vi "Do.vi"(8 "error in (no error)":errorcluster, 10 "Actor in":refnum<class "Actor.lvclass">, 11 "Update Energy Storage Parameter Msg":refnum<class "Update Energy Storage Parameter Msg.lvclass">) -> (0 "error out":errorcluster, 2 "Actor out":refnum<class "Actor.lvclass">)   [LabVIEW 2016, in "Optimization Framework.lvlib" / "Update Energy Storage Parameter Msg.lvclass"]
doc: "This VI delivers the message to the actor by calling the appropriate method(s) on the actor."
uses:
  Update Energy Storage Parameter Msg.lvclass
  <vilib>/ActorFramework/Actor/Actor.lvclass
  Optimization/Optimization.lvclass
  C:/Program Files (x86)/National Instruments/LabVIEW 2016/vi.lib/ActorFramework/Actor/Actor.lvclass
  Update Energy Storage Parameter Msg.lvclass/Update Energy Storage Parameter Msg.ctl
  Optimization/Optimization.lvclass/Optimization.ctl
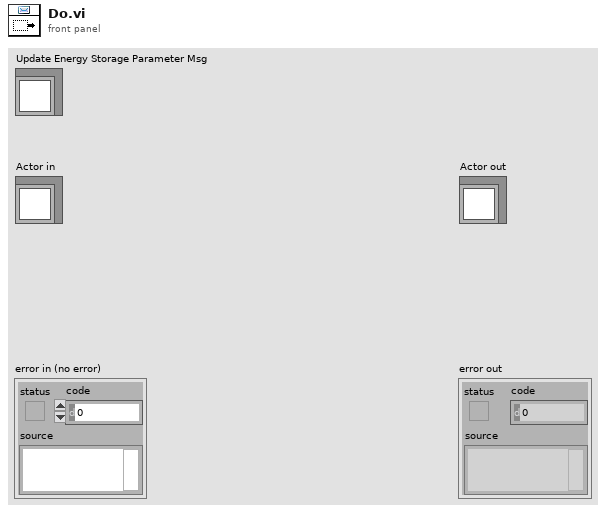
[diagram p1: front panel]
types:
  T1 = typedef "Optimization Framework.lvlib/Optimization.lvclass/Optimization Parameters Energy Storage.ctl" = cluster{"Device ID":u64, "Bus ID":u16, "Voltage (V)":dbl, "Power Rating (kVA)":dbl, "Energy Rating (kWh)":dbl, "Ramp Rate (kW/s)":dbl, "Max Power Factor (leading)":dbl, "Max Power Factor (lagging)":dbl, "Charging Efficiency Curve Power":dbl[], "Charging Efficiency Curve Efficiency":dbl[], "Discharging Efficiency Curve Power":dbl[], "Discharging Efficiency Curve Efficiency":dbl[], "Min SOC(%)":dbl, "Max SOC(%)":dbl, "Start SOC(%)":dbl, "End SOC(%)":dbl, "Control Capabilities":T2}
  T2 = typedef "Optimization Framework.lvlib/Optimization.lvclass/Device Control Capabilities.ctl" = cluster{"VF":bool, "P":bool, "Q":bool, "PF":bool, "PV":bool}
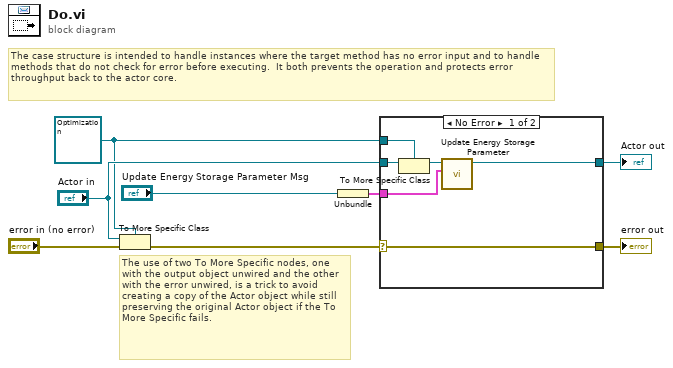
[diagram p0: block diagram]
diagram:
  w2 = refnum<class "Optimization.lvclass"> refnum ("Actor in")
  # "The use of two To More Specific nodes, one with the output object unwired and the other with the error unwired, is a trick to avoid creating a copy of the Actor object while still preserving the original Actor object if the To More Specific fails."
  # "The case structure is intended to handle instances where the target method has no error input and to handle methods that do not check for error before executing.  It both prevents the operation and protects error throughput back to the actor core."
  n1 = To More Specific Class(target class=w2, reference="Actor in", error in="error in (no error)") -> (error out=w6:errorcluster)  [unwired: 1 out]
  n2 = Unbundle("Update Energy Storage Parameter Msg") -> (w1:T1)
  n3 = case shown="No Error" w6 {
    selector: w6 -> [w13 w16]
    tunnel: [w13 w16] -> w5
    tunnel: [w14 w15] -> w4
    tunnel: "Actor in" -> [w12 w15]
    tunnel: w2 -> [w11 _]
    tunnel: w1 -> [w9 _]
    frame No Error {
      n4 = To More Specific Class(target class=w11, reference=w12) -> (specific class reference=w10:refnum<class "Optimization.lvclass">)  [unwired: 1 in, 1 out]
      n5 = call "Update Energy Storage Parameter.vi"("Energy Storage Parameters"=w9, "Optimization in"=w10) -> ("Optimization out"=w14:refnum<class "Optimization.lvclass">)  [unwired: 9 in]
    }
    frame Error {
      # "If type check fails, pass the original object out again."
    }
  }
  "error out" <- w5
  "Actor out" <- w4
